vi "Template.vi"(11 "jettl Msg Template in":refnum<class "jettl Msg Template.lvclass">) -> (3 "jettl Msg Template out":refnum<class "jettl Msg Template.lvclass">)   [LabVIEW 2021, in "_Template.lvlib" / "Templates.lvlib" / "jettl Msg Template.lvlib" / "jettl Msg Template.lvclass"]
uses:
  jettl Msg Template.lvclass
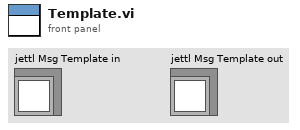
[diagram p1: front panel]
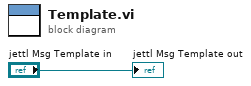
[diagram p0: block diagram]
diagram:
  "jettl Msg Template out" <- "jettl Msg Template in"
